vi "Set Pre and Post Build Actions.vi"(8 "error in (no error)":errorcluster, 9 "Post Build Action VI":refnum<vi>, 10 "Pre Build Action VI":refnum<vi>, 11 "Build in":refnum<class "NI_AB_API_Build.lvclass">) -> (0 "error out":errorcluster, 3 "Build out":refnum<class "NI_AB_API_Build.lvclass">)   [LabVIEW 2020, in "NI_AB_API_Build.lvclass"]
uses:
  <vilib>/AppBuilder/AB_API/Build/NI_AB_API_Build.lvclass
  <vilib>/AppBuilder/AB_API/Build/NI_AB_API_Build.lvclass/NI_AB_API_Build.ctl
  <vilib>/AppBuilder/AB_API/common/AB_API Build Action Type.ctl
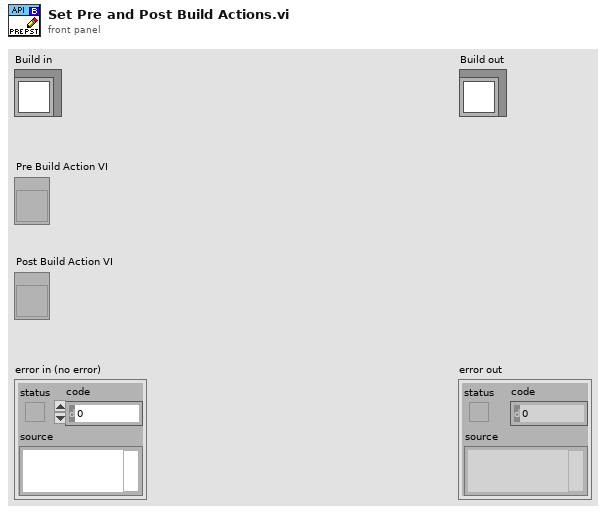
[diagram p1: front panel]
types:
  T1 = typedef "AB_API Build Action Type.ctl" = enum16{"Pre-Build", "Post-Build"}
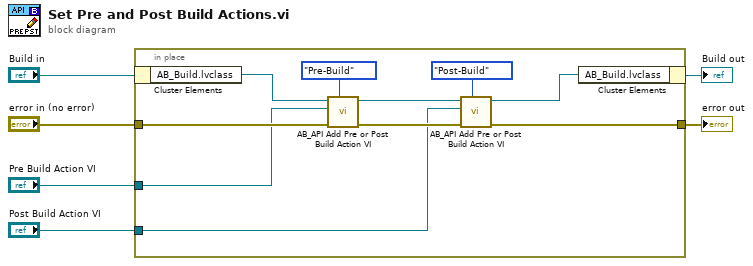
[diagram p0: block diagram]
diagram:
  n1 = in-place {
    in-place-border: "Pre Build Action VI" -> [w10]
    in-place-border: "error in (no error)" -> [w15]
    in-place-border: [w12] -> w2
    in-place-border: "Post Build Action VI" -> [w9]
    n2 = in-place-cluster #1("Build in") -> ("AB_Build.lvclass"=w16:refnum<class "AB_Build.lvclass">)
    n3 = call <vilib>:"AB_API Add Pre or Post Build Action VI.vi"("Action Type"=AB_API_Build_Action_Type."Pre-Build", "error in (no error)"=w15, "Action VI"=w10, "Build in"=w16) -> ("error out"=w14:errorcluster, "Build out"=w13:refnum<class "AB_Build.lvclass">)  [unwired: 6 in]
    n4 = call <vilib>:"AB_API Add Pre or Post Build Action VI.vi"("Action Type"=AB_API_Build_Action_Type."Post-Build", "error in (no error)"=w14, "Action VI"=w9, "Build in"=w13) -> ("error out"=w12:errorcluster, "Build out"=w11:refnum<class "AB_Build.lvclass">)  [unwired: 6 in]
    n5 = in-place-cluster #1("AB_Build.lvclass"=w11) -> (→"Build out":refnum<class "NI_AB_API_Build.lvclass">)
  }
  "error out" <- w2
